vi "ExecutionLoop-FrontPanelTemplate.vi"(8 "error in (no error)":errorcluster, 11 "Actor In":refnum<class>) -> (0 "error out":errorcluster, 3 "Actor Out":refnum<class>)   [LabVIEW 2017, in "LapDog.Messaging.v3.ActorTemplates.lvlib"]
uses:
  LapDog.Messaging.v3.ActorTemplates.lvlib
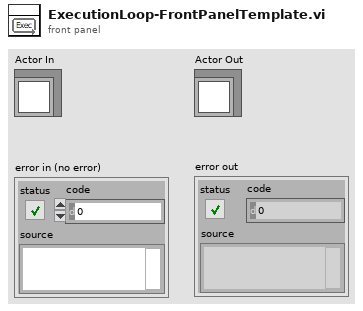
[diagram p1: front panel]
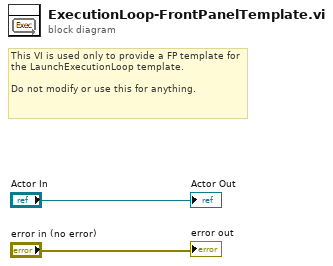
[diagram p0: block diagram]
diagram:
  # "This VI is used only to provide a FP template for the LaunchExecutionLoop template.\n\nDo not modify or use this for anything."
  "Actor Out" <- "Actor In"
  "error out" <- "error in (no error)"
